vi "Trap_Read_Wfm.vi"(8 "error in (no error)":errorcluster, 9 "Waveform Name":string="Adiabatic_RC_2_0_2000", 10 "Trapping Waveforms File Filter":string="*.bin", 11 "Trapping Waveforms Path":path=path "D:/PIRENEA/TRAPPING_WFMS") -> (0 "error out":errorcluster caption="sortie d'erreur", 2 "Wfm size":i32, 3 "Wfm data":dbl[](graph))   [LabVIEW 2020]
doc: "From a start and end value, generates an adiabatic waveform signal of 2000 values (double).\nWrites this waveform into a binary file, in a big-endian format.\nDisplays the written data and the FFT of the signal.\nDefault Path for the generated file is D:\\PIRENEA\\EXCIT_WFMS\n\nAvailable Waveforms : Sinus, Swift, Chirp, Ramp (Up or Down), DoubleRamp (Up-Down or Down-Up)"
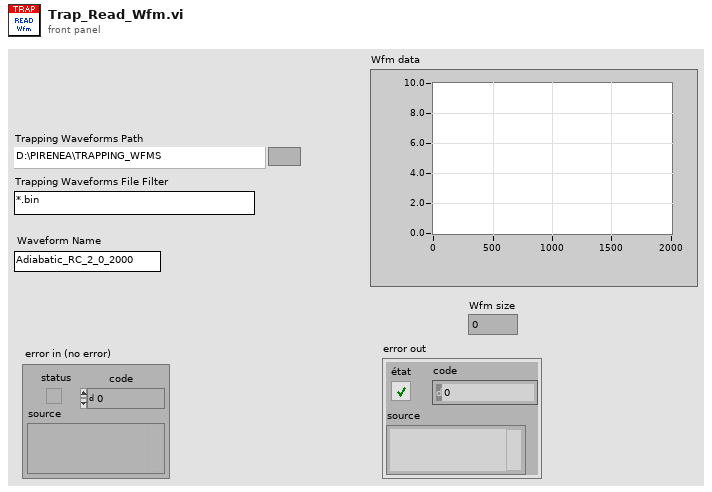
[diagram p1: front panel]
types:
  T1 = enum16{"big-endian, network order", "native, host order", "little-endian"}
  T2 = enum16{"open", "replace", "create", "open or create", "replace or create", "replace or create with confirmation"}
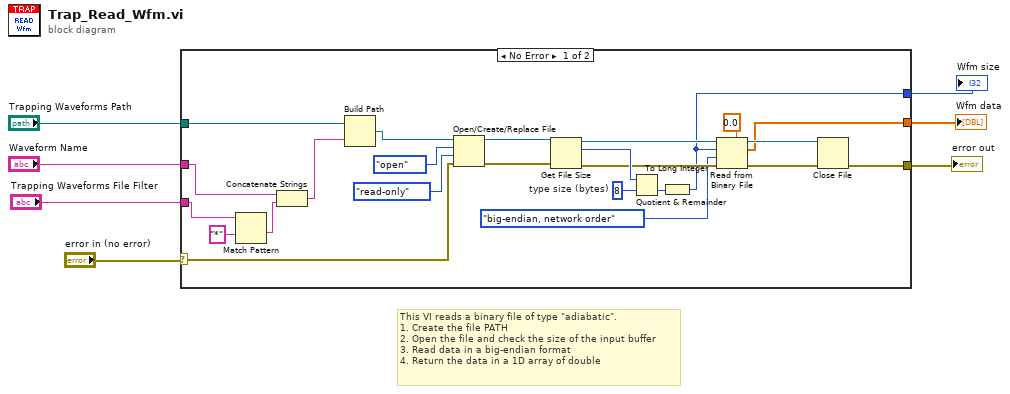
[diagram p0: block diagram]
diagram:
  # "This VI reads a binary file of type \"adiabatic\".\n1. Create the file PATH\n2. Open the file and check the size of the input buffer\n3. Read data in a big-endian format\n4. Return the data in a 1D array of double"
  n1 = case shown="No Error" "error in (no error)" {
    selector: "error in (no error)" -> [w15 w32]
    tunnel: [w14 w32] -> w7
    tunnel: "Trapping Waveforms Path" -> [w16 _]
    tunnel: "Trapping Waveforms File Filter" -> [w9 _]
    tunnel: "Waveform Name" -> [w18 _]
    tunnel: [w13 _] -> w2
    tunnel: [w11 _] -> w1
    frame No Error {
      w22 = i64 8  # type size (bytes)
      n2 = Match Pattern(string=w9, regular expression="*" ("expression régulière")) -> (after substring=w8:string)  [unwired: 1 in, 3 out]
      n3 = Concatenate Strings(w18, w8) -> (w17:string)
      n4 = Build Path(base path=w16, name or relative path=w17) -> (appended path=w19:path)
      n5 = Open/Create/Replace File(file path (use dialog)=w19, error in=w15, operation (0:open)=T2."open" ("opération (0 : open)"), access (0:read/write)=enum16{"read/write", "read-only", "write-only"}."read-only") -> (refnum out=w21:refnum<file>, error out=w20:errorcluster)  [unwired: 2 in, 1 out]
      n6 = Get File Size(file=w21, error in=w20) -> (refnum out=w29:refnum<file>, size (in bytes)=w26:i64, 0:w25:errorcluster)
      n7 = Quotient & Remainder(x=w26, y=w22) -> (floor(x/y)=w12:i64)  [unwired: 1 out]
      n8 = To Long Integer(number=w12) -> (32bit integer=w11:i32)
      n9 = Read from Binary File(5:0.0 ("data type"), 8:w25, 9:T1."big-endian, network order" ("byte order"), 10:w11, 11:w29) -> (0:w27:errorcluster, 2:w13:dbl[], 3:w28:refnum<file>)  [unwired: 1 in, 1 out]
      n10 = Close File(refnum=w28, error in=w27) -> (error out=w14:errorcluster)  [unwired: 1 out]
    }
    frame Error {
    }
  }
  "error out" <- w7
  "Wfm data" <- w2
  "Wfm size" <- w1
